vi "p10 decodificador de imagenes gris.vi"() -> ()   [LabVIEW 2013]
panel:
  in  "path to BMP file 3":path
  in  "path to BMP file":path
  in  "Array":bool[](array[boolean])
  out "new picture 2":picture
  out "new picture":picture
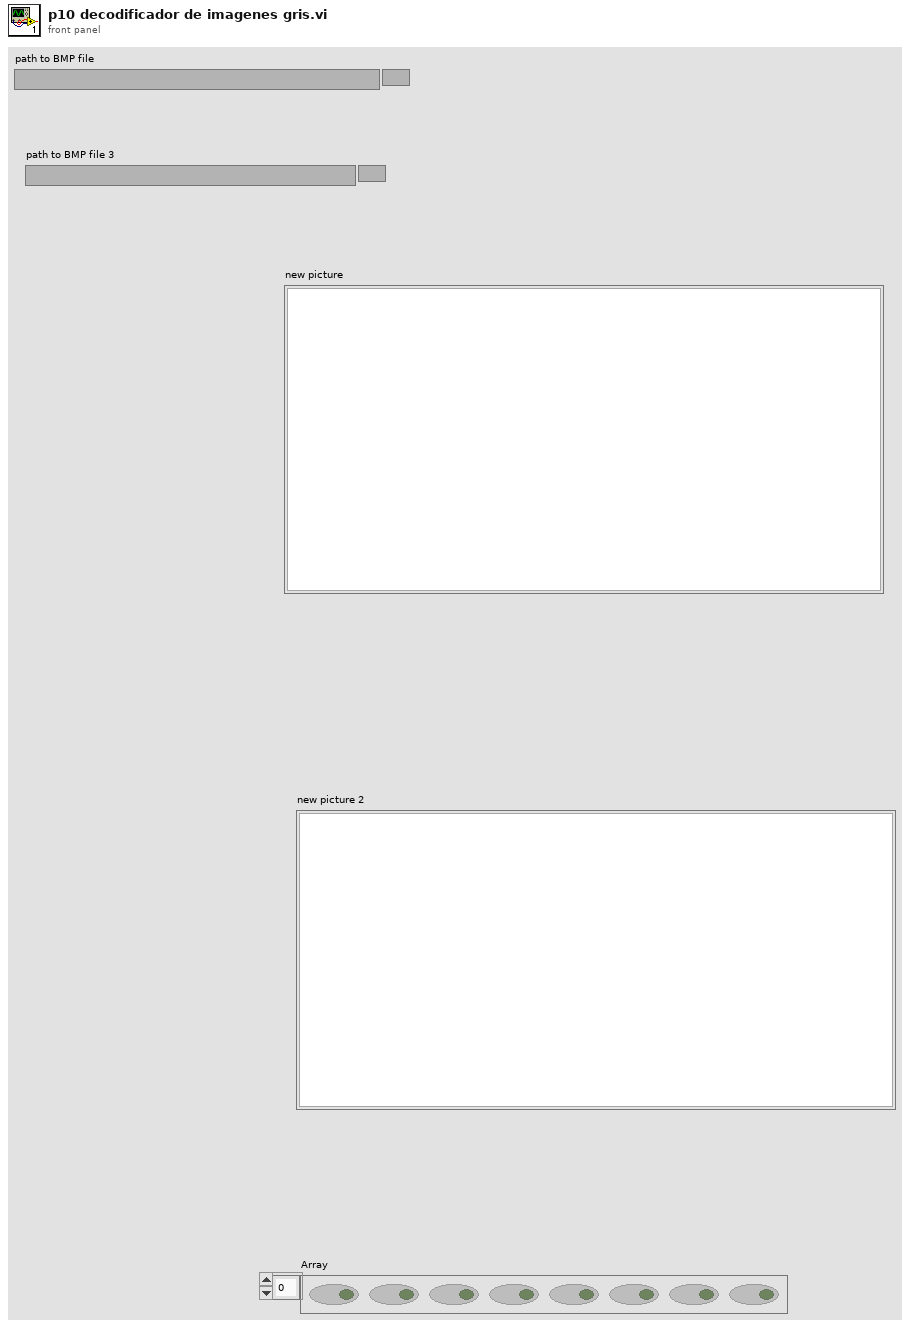
[diagram p1: front panel]
types:
  T1 = typedef "imagedata.ctl" = cluster{"image type":i32, "image depth":i32, "image":u8[], "mask":u8[], "colors":u32[], "Rectangle":cluster{"left":i16, "top":i16, "right":i16, "bottom":i16}}
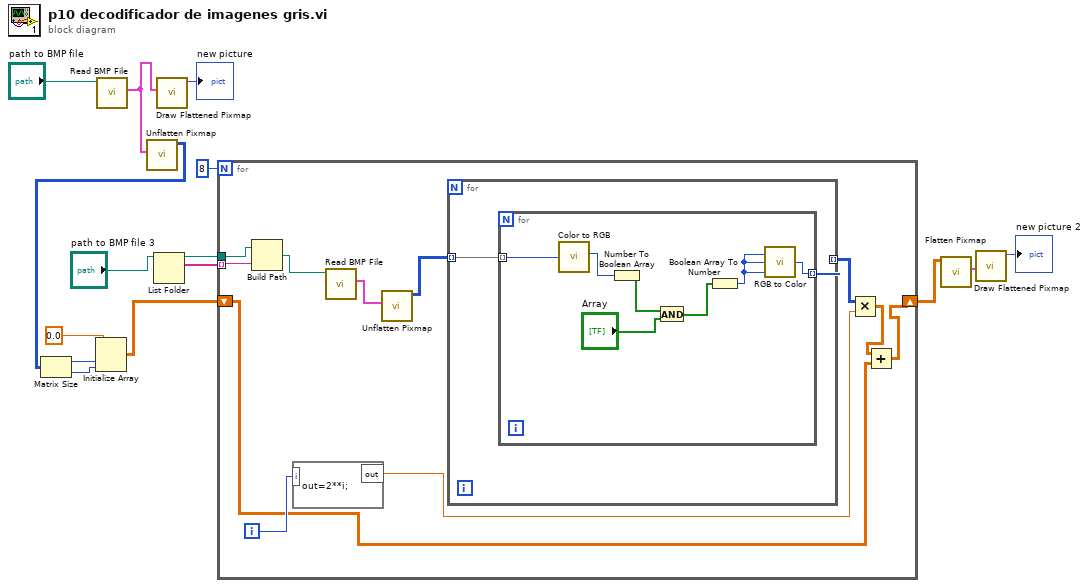
[diagram p0: block diagram]
diagram:
  n1 = call <vilib>:"Read BMP File.vi"("path to BMP file"="path to BMP file") -> ("image data"=w10:T1)  [unwired: 8 in, 2 out]
  n2 = call <vilib>:"Unflatten Pixmap.vi"("image data"=w10) -> ("24-bit pixmap"=w3:u32[][])  [unwired: 4 in, 6 out]
  n3 = Matrix Size(0:w3) -> (1:w2:i32, 2:w1:i32)
  n4 = Initialize Array(0.0 ("element"), w2, w1) -> (w4:dbl[][])
  n5 = List Folder(path="path to BMP file 3") -> (path out=w8:path, filenames=w7:string[])  [unwired: 3 in, 2 out]
  n6 = call <vilib>:"Draw Flattened Pixmap.vi"("image data"=w10) -> ("new picture"=→"new picture":picture)  [unwired: 8 in]
  n7 = for {
    N: 8 -> [_]
    tunnel: w8 -> [w22]
    tunnel: w7 -> [w21] mode=indexing
    shift-right: [w16] -> w6
    shift-left: w4 -> [w18]
    i -> [w24]
    n8 = Build Path(base path=w22, name or relative path=w21) -> (appended path=w20:path)
    n9 = formula code="out=2**i;"("i"=w24) -> ("out"=w23:dbl)
    n10 = call <vilib>:"Read BMP File.vi"("path to BMP file"=w20) -> ("image data"=w26:T1)  [unwired: 8 in, 2 out]
    n11 = call <vilib>:"Unflatten Pixmap.vi"("image data"=w26) -> ("24-bit pixmap"=w25:u32[][])  [unwired: 4 in, 6 out]
    n12 = for {
      tunnel: w25 -> [w28] mode=indexing
      tunnel: [w27] -> w19 mode=indexing
      n13 = for {
        tunnel: w28 -> [w31] mode=indexing
        tunnel: [w30] -> w27 mode=indexing
        n14 = call <vilib>:"Color to RGB.vi"("Color"=w31) -> ("R"=w35:u8)  [unwired: 3 out]
        n15 = Number To Boolean Array(number=w35) -> (Boolean array=w34:bool[])
        n16 = And(x=w34, y="Array") -> (x .and. y?=w32:bool[])
        n17 = Boolean Array To Number(Boolean array=w32) -> (number=w29:u32)
        n18 = call <vilib>:"RGB to Color.vi"("B"=w29, "G"=w29, "R"=w29) -> ("Color"=w30:u32)
      }
    }
    n19 = Multiply(x=w19, y=w23) -> (x*y=w17:dbl[][])
    n20 = Add ("Add.vi")(x=w17, y=w18) -> (x+y=w16:dbl[][])
  }
  n21 = call <vilib>:"Flatten Pixmap.vi"("24-bit pixmap"=w6) -> ("image data"=w14:T1)  [unwired: 10 in]
  n22 = call <vilib>:"Draw Flattened Pixmap.vi"("image data"=w14) -> ("new picture"=→"new picture 2":picture)  [unwired: 8 in]
